vi "Audio.Scale Waveform Based on Max Amplitude.vi"(10 "Max Amplitude":dbl=0.9, 11 "Wvfrm In":waveform(dbl)) -> (3 "Wvfrm Out":waveform(dbl))   [LabVIEW 2018]
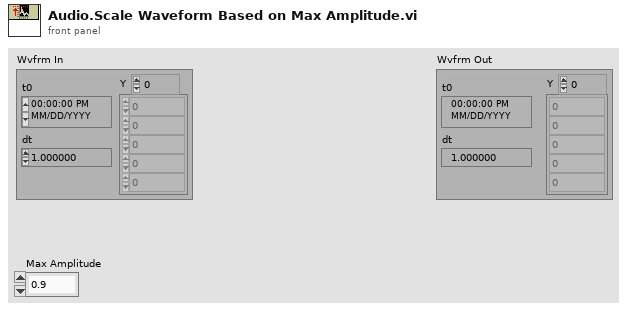
[diagram p1: front panel]
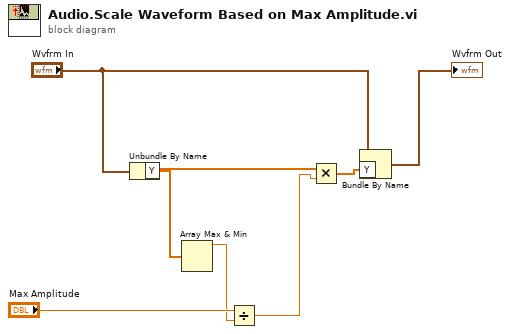
[diagram p0: block diagram]
diagram:
  n1 = Unbundle By Name("Wvfrm In") -> ("Y"=w3:dbl[])
  n2 = Array Max & Min(array=w3) -> (max value=w4:dbl)  [unwired: 3 out]
  n3 = Divide(x="Max Amplitude", y=w4) -> (x/y=w2:dbl)
  n4 = Multiply(x=w3, y=w2) -> (x*y=w1:dbl[])
  n5 = Bundle By Name(cluster="Wvfrm In", "Y"=w1) -> (→"Wvfrm Out":waveform(dbl))
